vi "Xc CURVE DETERMINATION.vi"(1 "Deslocamento X":dbl=7.0, 2 "Raio":dbl=7.0, 3 "Distância Ac (um)":dbl=50.0, 4 "Distância Guias (um)":dbl=50.0) -> (0 "Xc":dbl)   [LabVIEW 2014]
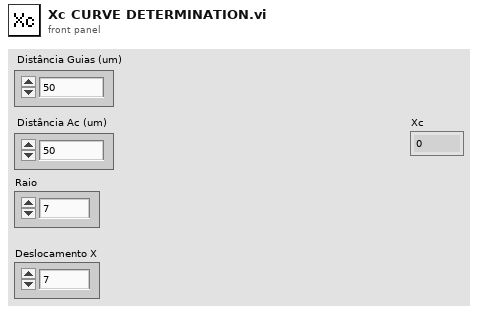
[diagram p1: front panel]
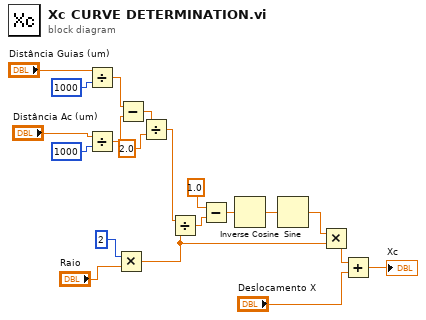
[diagram p0: block diagram]
diagram:
  n1 = Divide(x="Distância Guias (um)", y=1000) -> (x/y=w11:dbl)
  n2 = Divide(x="Distância Ac (um)", y=1000) -> (x/y=w10:dbl)
  n3 = Multiply(x=2 ("y"), y="Raio") -> (x*y=w5:dbl)
  n4 = Subtract(x=w11, y=w10) -> (x-y=w9:dbl)
  n5 = Divide(x=w9, y=2.0) -> (x/y=w7:dbl)
  n6 = Divide(x=w7, y=w5) -> (x/y=w16:dbl)
  n7 = Subtract(x=1.0, y=w16) -> (x-y=w18:dbl)
  n8 = Inverse Cosine(1:w18) -> (0:w19:dbl)
  n9 = Sine(x=w19) -> (sin(x)=w4:dbl)
  n10 = Multiply(x=w4, y=w5) -> (x*y=w3:dbl)
  n11 = Add(x=w3, y="Deslocamento X") -> (x+y=→"Xc":dbl)
